vi "CLFNSetPath.vi"(5 "New Path":path=path "gartoolkit_32-1.dll", 8 "error in (no error)":errorcluster, 11 "Files":path[](array[path])) -> (0 "error out":errorcluster, 3 "Unused Binaries":path[](array[path]))   [LabVIEW 2020]
uses:
  <vilib>/Utility/miscctls.llb/LVMapReplaceAction.ctl
  <vilib>/Utility/traverseref.llb/TRef TravTarget.ctl
  f7d54ce6-af0d-4369-8e73-8cd4f8e29281.vi
  <vilib>/Comparison/Less/Less Functor/Less Functor.lvclass
  <vilib>/Utility/traverseref.llb/VI Scripting - Traverse.lvlib
panel:
  out "Array":path[](array[path])
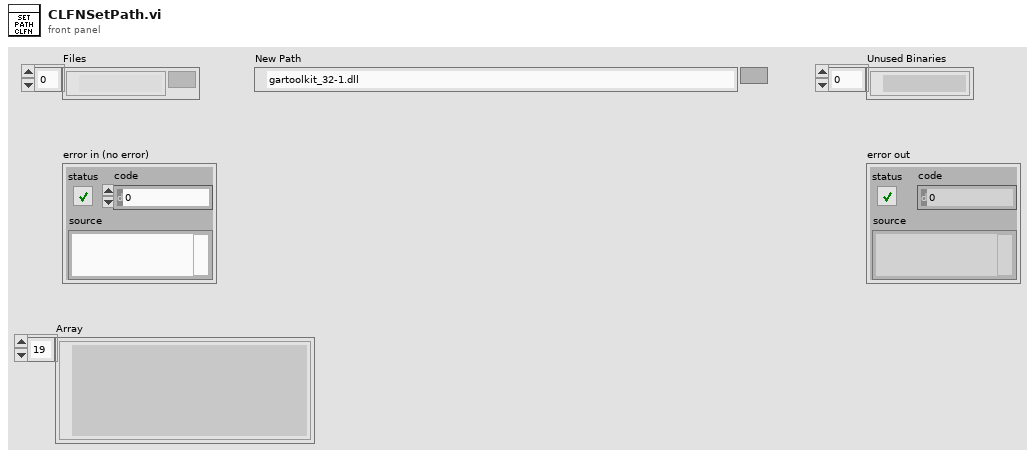
[diagram p1: front panel]
types:
  T1 = typedef "LVMapReplaceAction.ctl" = enum32{"Modify Entry only if found", "Add or Modify Entry", "Delete Entry"}
  T2 = typedef "TRef TravTarget.ctl" = enum16{"FP", "BD", "Other"}
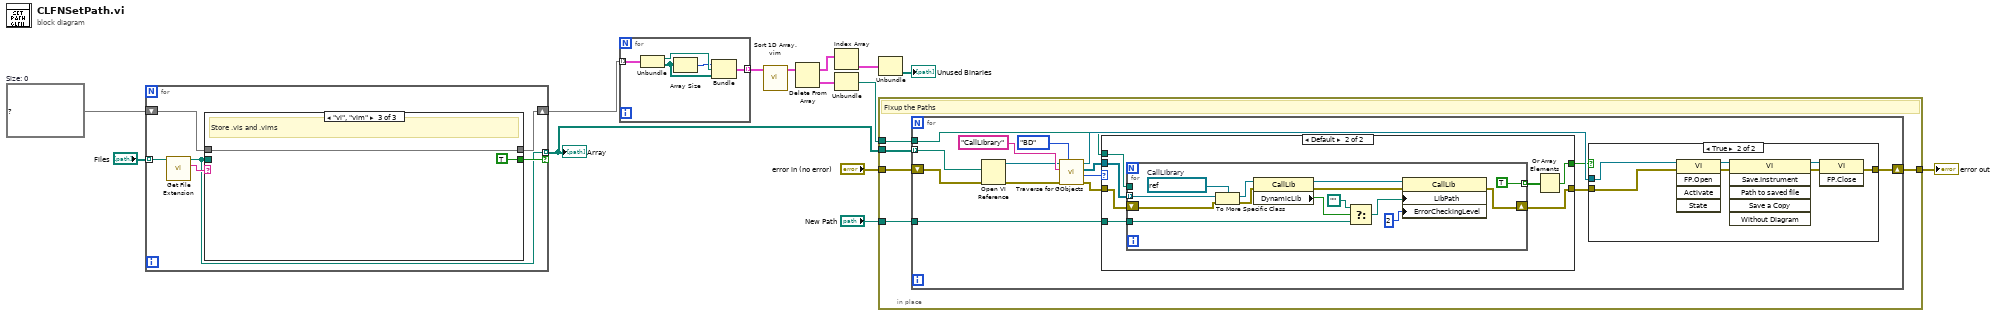
[diagram p0: block diagram]
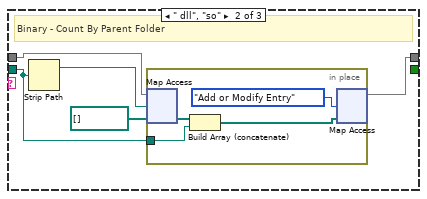
[diagram p3: hidden frame]
diagram:
  w14 = map{path, path[]} {}  # Size: 0
  n1 = for {
    tunnel: "Files" -> [w20] mode=indexing
    tunnel: [w17] -> w8 mode=indexing if=w18
    shift-right: [w16] -> w9
    shift-left: w14 -> [w15]
    n2 = call <vilib>:"Get File Extension.vi"("file"=w20) -> ("lowercase file extension"=w19:string, "dup file"=w17:path)  [unwired: 6 in, 3 out]
    n3 = case shown="\"vi\", \"vim\"" w19 {
      tunnel: [_ _ TRUE] -> w18
      tunnel: w17 -> [_ w22 _]
      tunnel: [w21 w24 w31] -> w16
      tunnel: w15 -> [w21 w23 w31]
      frame Default {
      }
      frame " dll", "so" {
        # "Binary - Count By Parent Folder"
        n4 = Strip Path(path=w22) -> (stripped path=w26:path)  [unwired: 1 out]
        n5 = in-place {
          in-place-border: w22 -> [w28]
          n6 = in-place-map #1(w23, w26, path[] []) -> (w29:path[])  [unwired: 1 out]
          n7 = Build Array (concatenate)(w29, w28) -> (w27:path[])
          n8 = in-place-map #1(w27, LVMapReplaceAction."Add or Modify Entry" ("action")) -> (w24:map{path, path[]})  [unwired: 2 out]
        }
      }
      frame "vi", "vim" {
        # "Store .vis and .vims"
      }
    }
  }
  "Array" <- w8
  n9 = for {
    tunnel: w9 -> [w37] mode=indexing
    tunnel: [w35] -> w10 mode=indexing
    n10 = Unbundle(w37) -> ("stripped path"=w36:path, w33:path[])
    n11 = Array Size(array=w33) -> (size(s)=w34:i32)
    n12 = Bundle(w34, "stripped path"=w36, w33) -> (w35:cluster{i32, "stripped path":path, path[]})  [unwired: 1 in]
  }
  n13 = call "Sort 1D Array.vim"("unsorted array"=w10) -> ("sorted array"=w11:cluster{i32, "stripped path":path, path[]}[])  [unwired: 10 in]
  n14 = Delete From Array(array=w11) -> (deleted portion=w12:cluster{i32, "stripped path":path, path[]}, array with subset deleted=w4:cluster{i32, "stripped path":path, path[]}[])  [unwired: 2 in]
  n15 = Index Array(array=w4) -> (element=w3:cluster{i32, "stripped path":path, path[]})  [unwired: 1 in]
  n16 = Unbundle(w12) -> ("stripped path"=w13:path)  [unwired: 2 out]
  n17 = Unbundle(w3) -> (→"Unused Binaries":path[])  [unwired: 2 out]
  n18 = in-place {
    in-place-border: [w39] -> w6
    in-place-border: w8 -> [w42]
    in-place-border: w13 -> [w41]
    in-place-border: "error in (no error)" -> [w40]
    in-place-border: "New Path" -> [w38]
    # "Fixup the Paths"
    n19 = for {
      tunnel: w42 -> [w55] mode=indexing
      shift-right: [w53] -> w39
      shift-left: w40 -> [w52]
      tunnel: w41 -> [w45]
      tunnel: w38 -> [w44]
      n20 = Open VI Reference(vi path=w55, error in (no error)=w52) -> (vi reference=w48:refnum<vi>, error out=w47:errorcluster)  [unwired: 4 in]
      n21 = call <vilib>:"Traverse for GObjects.vi"("Traverse Target"=TRef_TravTarget."BD", "error in (no error)"=w47, "Class Name"="CallLibrary", "VI Refnum"=w48) -> ("error out"=w51:errorcluster, "# of Refs"=w43:i32, "References"=w46:refnum<vi>[], "dup VI Refnum"=w57:refnum<vi>)  [unwired: 4 in]
      n22 = case shown="Default" w43 {
        tunnel: [w58 w65] -> w56
        tunnel: [_ w64] -> w54
        tunnel: w51 -> [w58 w63]
        tunnel: w46 -> [_ w62]
        tunnel: w45 -> [_ w60]
        tunnel: w44 -> [_ w59]
        frame 0 {
        }
        frame Default {
          n23 = for {
            tunnel: w62 -> [w72] mode=indexing
            shift-right: [w79] -> w65
            shift-left: w63 -> [w74]
            tunnel: [TRUE] -> w61 mode=indexing
            tunnel: w60 -> [_]
            tunnel: w59 -> [w69]
            w73 = refnum<vi> refnum  # CallLibrary
            n24 = To More Specific Class(target class=w73, reference=w72, error in=w74) -> (specific class reference=w75:refnum<vi>, error out=w76:errorcluster)
            n25 = property class="CallLib"(reference=w75, error in=w76) -> (reference out=w78:refnum<vi>, error out=w77:errorcluster, "DynamicLib"=w70:bool)
            n26 = Select(t=path "", s=w70, f=w69) -> (s? t:f=w68:path)
            n27 = property class="CallLib"(reference=w78, error in=w77, "LibPath"=w68, "ErrorCheckingLevel"=u32 2 ("Error Checking Level")) -> (error out=w79:errorcluster)  [unwired: 1 out]
          }
          n28 = Or Array Elements(Boolean array=w61) -> (logical OR=w64:bool)
        }
      }
      n29 = case shown="True" w54 {
        tunnel: w57 -> [_ w82]
        tunnel: w56 -> [w80 w81]
        tunnel: [w80 w86] -> w53
        frame False {
        }
        frame True {
          n30 = invoke class="VI" method="FP.Open"(reference=w82, error in=w81) -> (reference out=w84:refnum<vi>, error out=w83:errorcluster)  [unwired: 3 in, 3 out]
          n31 = invoke class="VI" method="Save.Instrument"(reference=w84, error in=w83) -> (reference out=w85:refnum<vi>, error out=w87:errorcluster)  [unwired: 4 in, 4 out]
          n32 = invoke class="VI" method="FP.Close"(reference=w85, error in=w87) -> (error out=w86:errorcluster)  [unwired: 1 in, 2 out]
        }
      }
    }
  }
  "error out" <- w6
